vi "Lian_Lab05_I.vi"() -> ()   [LabVIEW 2020]
uses:
  <vilib>/express/express analysis/Spectral/Block/exnSpectralBlock spectral measurements peak poly.vi
  <vilib>/express/express analysis/Spectral/Block/exnSpectralBlock spectral measurements peak DDT.vi
  <vilib>/express/express analysis/Spectral/XNode/ExpressSpectralMeasurementsBlockNode.xnode
panel:
  out "Iterations":i32
  in  "?":bool
  out "Waveform Graph":dynamicdata(graph)
  out "Acceleration":dynamicdata(graph)
  out "Raw Voltage":dynamicdata(graph)
  in  "number of samples":i32=50
  in  "sampling rate":dbl=1000.0
  # "Fundamental Frequency Measurement"
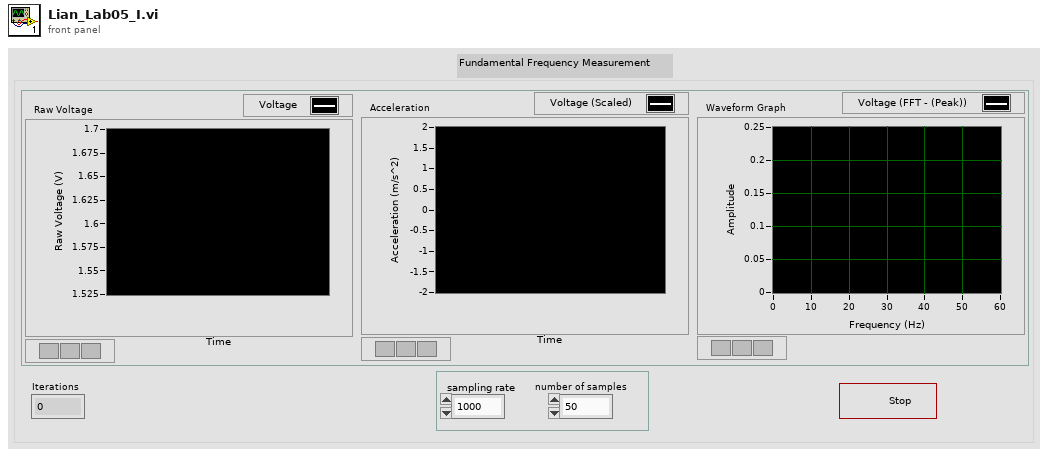
[diagram p1: front panel]
types:
  T1 = cluster{"averaging mode":u16, "weighting mode":u16, "number of averages":u32}
  T2 = cluster{"dB On (F)":bool, "unwrap phase (F)":bool, "convert to degree (F)":bool}
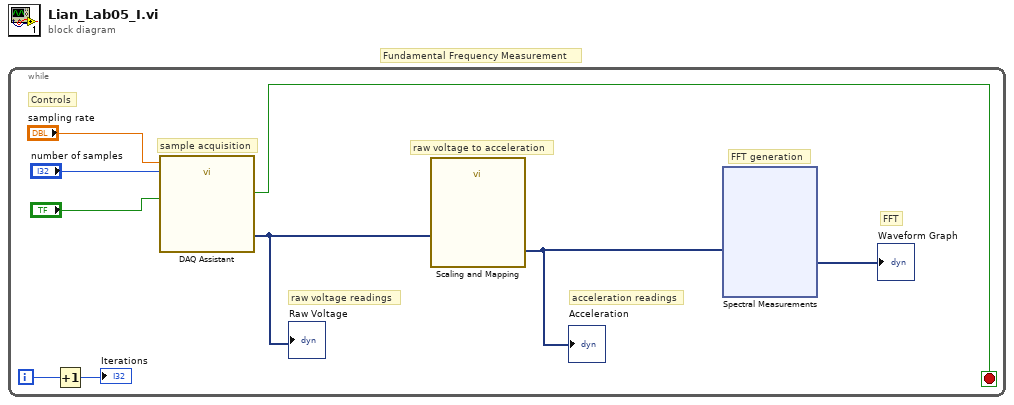
[diagram p0: block diagram]
diagram:
  # "Fundamental Frequency Measurement"
  n1 = while {
    i -> [w2]
    stop <- w3 stop-if-true
    # "FFT"
    # "Controls"
    # "FFT generation"
    # "sample acquisition"
    # "raw voltage to acceleration"
    # "acceleration readings"
    # "raw voltage readings"
    n2 = Increment(x=w2) -> (x+1=→"Iterations":i32)
    n3 = call "DAQ Assistant"("rate"="sampling rate", "number of samples"="number of samples", "stop (F)"="?") -> ("data"=w7:dynamicdata, "stopped"=w3:bool)  [unwired: 13 in, 2 out]
    "Raw Voltage" <- w7
    n4 = call "Scaling and Mapping"("Signals"=w7) -> ("Scaled Signals"=w4:dynamicdata)  [unwired: 9 in, 1 out]
    "Acceleration" <- w4
    n5 = xnode "Spectral Measurements"("Signals"=w4) -> ("FFT - (Peak)"=→"Waveform Graph":dynamicdata)  [unwired: 1 in, 2 out]
  }
